vi "generate full tag select table.vi"(7 "Full Alarms Table":refnum<vi>, 8 "error in":errorcluster, 10 "engine configuration":refnum<class "engine configuration.lvclass">, 11 "tag bus configurable plugin module configuration":refnum<class "tag select module configuration.lvclass">) -> (0 "error out":errorcluster)   [LabVIEW 2013, in "tag select module editor node.lvclass"]
uses:
  tag select module editor node.lvclass
  module/configuration/tag select module configuration.lvclass
  <vilib>/NI/Module Execution Interface/Engine Configuration/engine configuration.lvclass
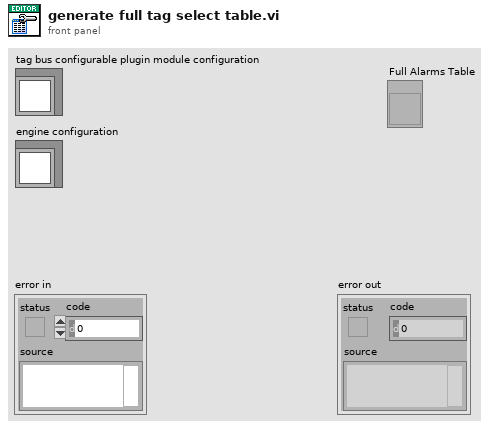
[diagram p1: front panel]
types:
  T1 = typedef "tag select module configuration.lvclass/tag select configuration.ctl" = cluster{"tag select name":string, "data type":T2, "output":refnum<class "TBM channel.lvclass">, "select":refnum<class "TBM channel.lvclass">, "input channels":refnum<class "TBM channel.lvclass">[]}
  T2 = typedef "tag bus.lvlib/tag descriptor.lvclass/Data Type.ctl" = enum16{"Double", "Single", "I64", "I32", "I16", "I8", "U64", "U32", "U16", "U8", "Boolean", "String", "Array of Double", "Array of Single", "Array of I64", "Array of I32", "Array of I16", "Array of I8", "Array of U64", "Array of U32", "Array of U16", "Array of U8", "Array of Boolean", "Array of String"}
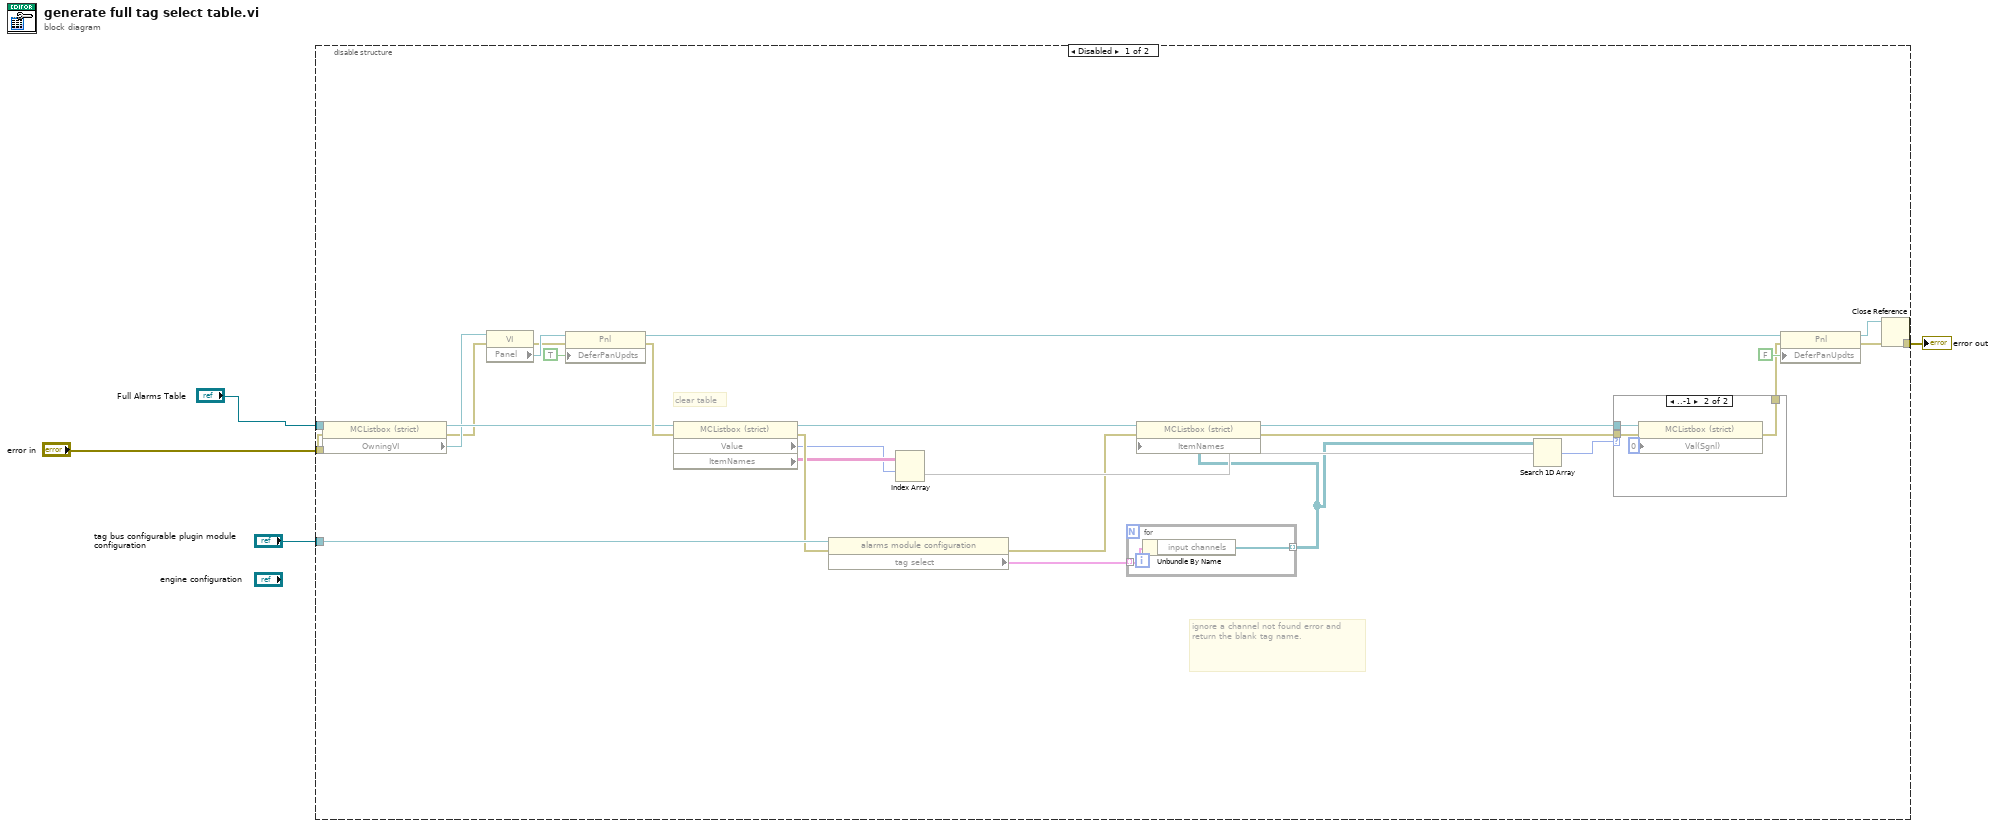
[diagram p0: block diagram]
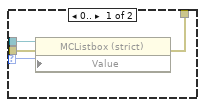
[diagram p2: hidden frame]
diagram:
  n1 = disable-structure shown="Disabled" {
    disable-tunnel: "tag bus configurable plugin module configuration" -> [w31 _]
    disable-tunnel: "error in" -> [w19 w42]
    disable-tunnel: [w16 w42] -> w2
    disable-tunnel: "Full Alarms Table" -> [w5 _]
    frame Disabled {
      # "ignore a channel not found error and return the blank tag name."
      # "clear table"
      n2 = property class="MCListbox (strict)"(reference=w5, error in=w19) -> (reference out=w20:refnum<vi>, error out=w17:errorcluster, "OwningVI"=w18:refnum<vi>)
      n3 = property class="VI"(reference=w18, error in=w17) -> (error out=w26:errorcluster, "Panel"=w27:refnum<vi>)  [unwired: 1 out]
      n4 = property class="Pnl"(reference=w27, error in=w26, "DeferPanUpdts"=TRUE ("Defer Panel Updates")) -> (reference out=w23:refnum<vi>, error out=w25:errorcluster)
      n5 = property class="MCListbox (strict)"(reference=w20, error in=w25) -> (reference out=w10:refnum<vi>, error out=w29:errorcluster, "Value"=w13:i32, "ItemNames"=w14:string[][])
      n6 = property class="alarms module configuration"(reference=w31, error in=w29) -> (error out=w8:errorcluster, "tag select"=w30:T1[])  [unwired: 1 out]
      n7 = Index Array(array=w14, index (row)=w13) -> (element=w11:string[])  [unwired: 1 in]
      n8 = for {
        tunnel: w30 -> [w33] mode=indexing
        tunnel: [w32] -> w6 mode=indexing
        n9 = Unbundle By Name(w33) -> ("input channels"=w32:refnum<class "TBM channel.lvclass">[])
      }
      n10 = property class="MCListbox (strict)"(reference=w10, error in=w8, "ItemNames"=w6) -> (reference out=w9:refnum<vi>, error out=w7:errorcluster)
      n11 = Search 1D Array(1D array=w6, element=w11) -> (index of element=w12:i32)  [unwired: 1 in]
      n12 = case shown="..-1" w12 {
        selector: w12 -> [w34 _]
        tunnel: w9 -> [w37 w41]
        tunnel: w7 -> [w36 w40]
        tunnel: [w35 w39] -> w22
        frame 0.. {
          n13 = property class="MCListbox (strict)"(reference=w37, error in=w36, "Value"=w34) -> (error out=w35:errorcluster)  [unwired: 1 out]
        }
        frame ..-1 {
          n14 = property class="MCListbox (strict)"(reference=w41, error in=w40, "Val(Sgnl)"=0 ("Value (Signaling)")) -> (error out=w39:errorcluster)  [unwired: 1 out]
        }
      }
      n15 = property class="Pnl"(reference=w23, error in=w22, "DeferPanUpdts"=FALSE ("Defer Panel Updates")) -> (reference out=w15:refnum<vi>, error out=w21:errorcluster)
      n16 = Close Reference(reference=w15, error in (no error)=w21) -> (error out=w16:errorcluster)
    }
    frame Enabled {
    }
  }
  "error out" <- w2
